vi "VILab.vi"() -> ()   [LabVIEW 2023, in "VILab.lvlib"]
uses:
  VILab.lvlib
  Support Files/VILab/VILab Data.ctl
  Support Files/VILab/Attribute.lvclass
  Resource Manipulation/Resource Array.ctl
  Resource Manipulation/Resource.ctl
  Support Files/VILab/Tree Manager.lvclass
  Support Files/VILab/State Enum.ctl
  Resource Manipulation/Decompose VI (Refnum).vi
  Support Files/VILab/Data Item.lvclass
  Resource Manipulation.lvlib
panel:
  in  "Dissect":bool
  in  "Rebuild":bool
  in  "Properties":bool
  in  "Clone":bool
  in  "Delete":bool
  in  "Add":bool
  in  "Tree":string(tree)
  # "WARNING:\nThis unofficial utility has NO WARRANTY and uses internal LabVIEW functionality that is NOT supported by National Instruments.\nYou will very likely crash LabVIEW and create insane/corrupted VI's, so use this at your own risk. But that's all part of the Fun™, right? ;)"
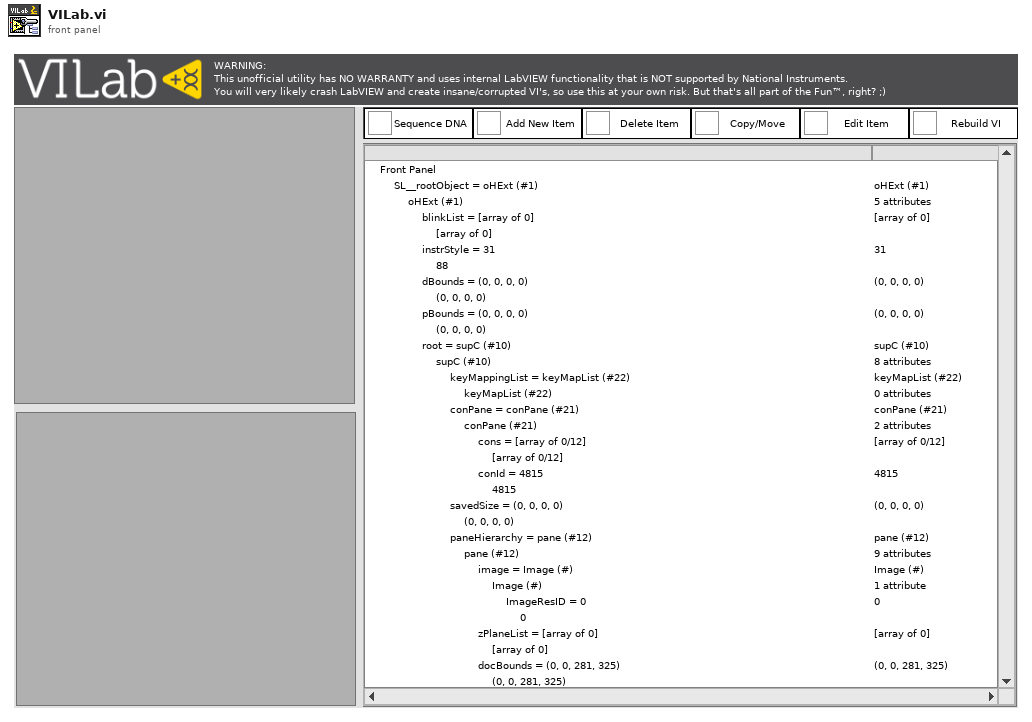
[diagram p1: front panel]
types:
  T1 = typedef "VILab.lvlib/State Enum.ctl" = enum16{"Initialize", "Event Handler", "Exit", "Edit Selected Item", "Dissect VI", "Rebuild VI"}
  T2 = typedef "VILab.lvlib/VILab Data.ctl" = cluster{"Embedded VI":refnum<vi>, "FP Root":refnum<class "Attribute.lvclass">, "BD Root":refnum<class "Attribute.lvclass">, "Def VI Res":T3, "Tree Mgr":refnum<class "Tree Manager.lvclass">}
  T3 = typedef "Resource Manipulation.lvlib/Resource Array.ctl" = T4[]
  T4 = typedef "Resource Manipulation.lvlib/Resource.ctl" = cluster{"type":u32, "id":i32, "name":string, "binary data":string}
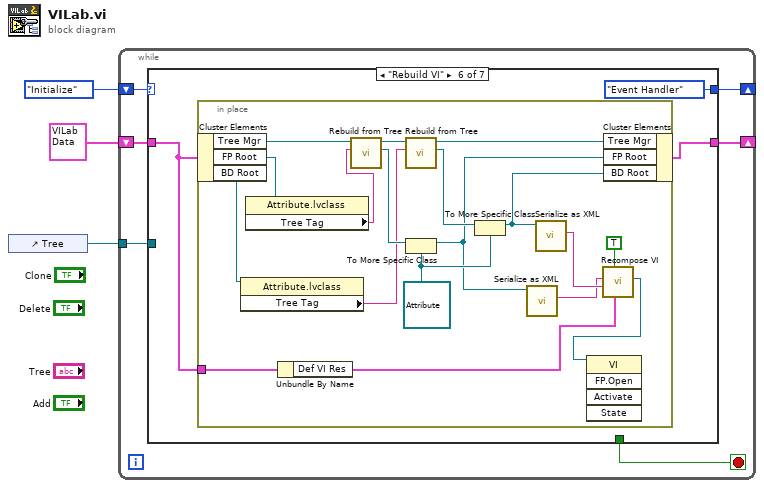
[diagram p0: block diagram]
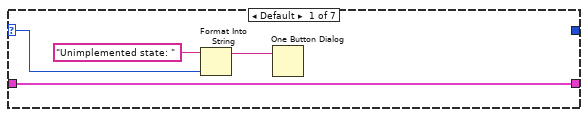
[diagram p2: hidden frame]
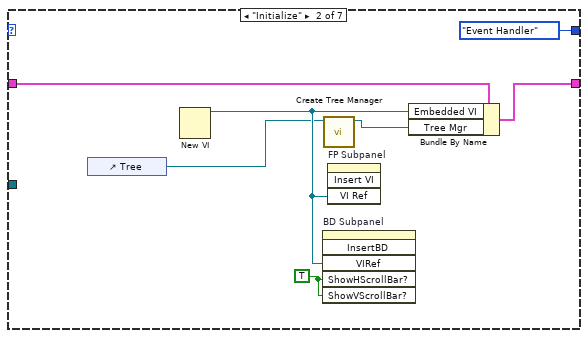
[diagram p3: hidden frame]
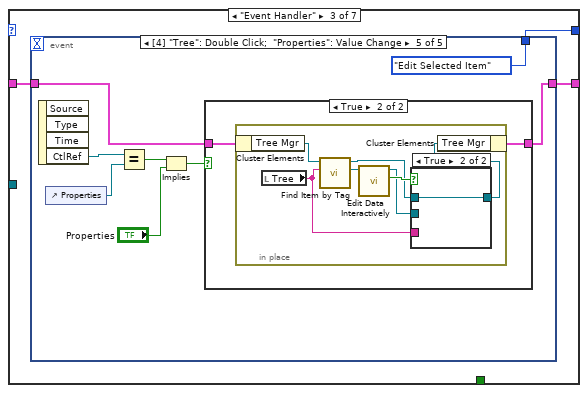
[diagram p4: hidden frame]
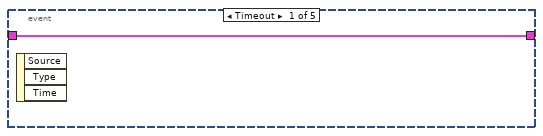
[diagram p5: hidden frame]
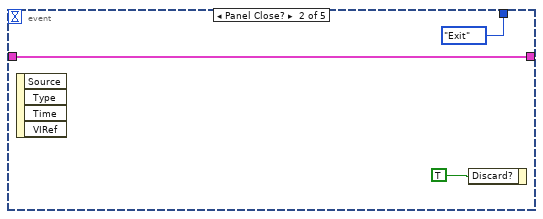
[diagram p6: hidden frame]
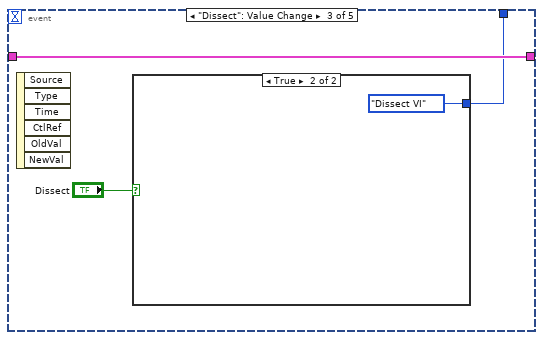
[diagram p7: hidden frame]
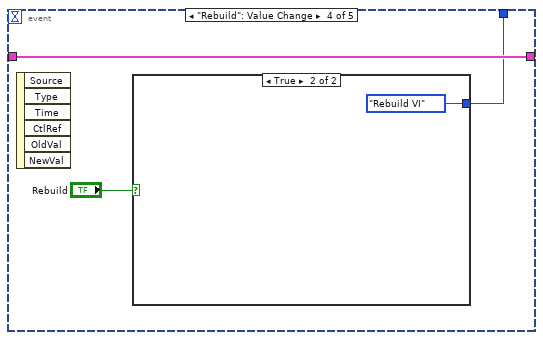
[diagram p9: hidden frame]
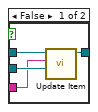
[diagram p12: hidden frame]
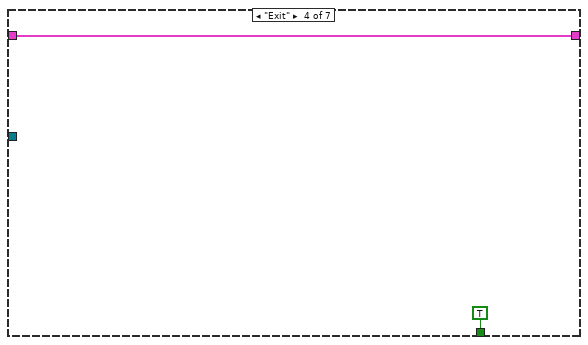
[diagram p13: hidden frame]
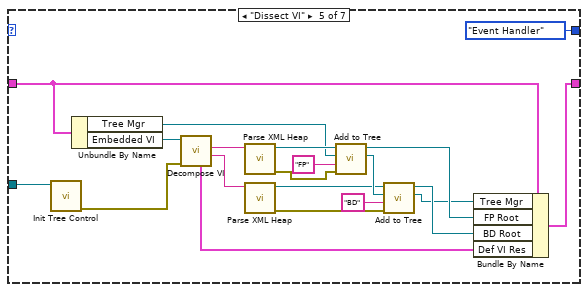
[diagram p14: hidden frame]
diagram:
  n1 = control-ref of="Tree"() -> (w1:refnum<vi>)
  n2 = while {
    shift-right: [w6] -> _
    shift-left: State_Enum."Initialize" ("State") -> [w9]
    shift-right: [w7] -> _
    shift-left: T2 {"Embedded VI"=refnum, "FP Root"=refnum, "BD Root"=refnum, "Def VI Res"=[], "Tree Mgr"=refnum} ("Data") -> [w8]
    tunnel: w1 -> [w4]
    stop <- w5 stop-if-true
    n3 = case shown="\"Rebuild VI\"" w9 {
      selector: w9 -> [w11 _ _ _ _ _ _]
      tunnel: w8 -> [w13 w20 w22 w60 w78 w81 w102]
      tunnel: [w13 w19 w23 w60 w76 w82 w102] -> w7
      tunnel: [_ State_Enum."Event Handler" ("State") w21 _ State_Enum."Event Handler" ("State") State_Enum."Event Handler" ("State") _] -> w6
      tunnel: [_ _ _ TRUE ("Discard?") _ _ _] -> w5
      tunnel: w4 -> [_ _ _ _ w65 _ _]
      frame Default {
        n4 = Format Into String(initial string="Unimplemented state: ", w11) -> (resulting string=w10:string)  [unwired: 2 in, 1 out]
        n5 = One Button Dialog(message=w10) -> ()  [unwired: 1 in, 1 out]
      }
      frame "Initialize" {
        w18 = TRUE ("ShowHScrollBar")
        n6 = control-ref of="Tree"() -> (w14:refnum<vi>)
        n7 = New VI() -> (3:w17:refnum<vi>)  [unwired: 7 in, 1 out]
        n8 = invoke on="BD Subpanel" class="SubPnl" method="InsertBD"("VIRef"=w17, "ShowHScrollBar?"=w18, "ShowVScrollBar?"=w18) -> ()  [unwired: 3 in, 6 out]
        n9 = call "Create Tree Manager.vi"("Tree Control"=w14) -> ("Tree Manager"=w15:refnum<class "Tree Manager.lvclass">)  [unwired: 9 in, 1 out]
        n10 = invoke on="FP Subpanel" class="SubPnl" method="Insert VI"("VI Ref"=w17) -> ()  [unwired: 3 in, 4 out]
        n11 = Bundle By Name(cluster=w20, "Embedded VI"=w17, "Tree Mgr"=w15) -> (w19:T2)
      }
      frame "Event Handler" {
        n12 = event shown="[4] \"Tree\": Double Click;  \"Properties\": Value Change" {
          selector: _ -> [_ _ _ _ _]
          dyn-events: _ -> [_ _ _ _ _]
          timeout: _ -> [_ _ _ _ _]
          tunnel: [w24 w27 w30 w34 w36] -> w23
          tunnel: w22 -> [w24 w27 w30 w34 w37]
          tunnel: [_ State_Enum."Exit" ("State") w28 w33 State_Enum."Edit Selected Item" ("State")] -> w21
          event Timeout {
            n13 = event-data() -> ()  [unwired: 1 in, 3 out]
          }
          event Panel Close? {
            n14 = event-data() -> ()  [unwired: 1 in, 4 out]
            n15 = event-data("Discard?"=TRUE) -> ()  [unwired: 1 in, 1 out]
          }
          event "Dissect": Value Change {
            n16 = event-data() -> ()  [unwired: 1 in, 6 out]
            n17 = case shown="True" "Dissect" {
              tunnel: [_ State_Enum."Dissect VI" ("State")] -> w28
              frame False {
              }
              frame True {
              }
            }
          }
          event "Rebuild": Value Change {
            n18 = event-data() -> ()  [unwired: 1 in, 6 out]
            n19 = case shown="True" "Rebuild" {
              tunnel: [_ State_Enum."Rebuild VI" ("State")] -> w33
              frame False {
              }
              frame True {
              }
            }
          }
          event "Tree": Double Click; "Properties": Value Change {
            n20 = event-data() -> ("CtlRef"=w42:refnum<vi>)  [unwired: 1 in, 3 out]
            n21 = control-ref of="Properties"() -> (w41:refnum<vi>)
            n22 = Equal?(x=w42, y=w41) -> (x = y?=w40:bool)
            n23 = Implies(1:"Properties", 2:w40) -> (0:w38:bool)
            n24 = case shown="True" w38 {
              tunnel: w37 -> [w44 w46]
              tunnel: [w44 w45] -> w36
              frame False {
              }
              frame True {
                n25 = in-place {
                  n26 = in-place-cluster #1(w46) -> ("Tree Mgr"=w52:refnum<class "Tree Manager.lvclass">)
                  n27 = local read "Tree"() -> (w47:string)
                  n28 = call "Find Item by Tag.vi"("Tag"=w47, "Tree Manager in"=w52) -> ("Data Item"=w53:refnum<class "Data Item.lvclass">, "Tree Manager out"=w49:refnum<class "Tree Manager.lvclass">)  [unwired: 6 in, 2 out]
                  n29 = call-dynamic "Edit Data Interactively.vi"("Data Item in"=w53) -> ("Cancel?"=w51:bool, "Data Item out"=w50:refnum<class "Data Item.lvclass">)  [unwired: 8 in, 1 out]
                  n30 = case shown="True" w51 {
                    tunnel: w50 -> [w57 _]
                    tunnel: w49 -> [w56 w58]
                    tunnel: [w55 w58] -> w48
                    tunnel: w47 -> [w54 _]
                    frame False {
                      n31 = call "Update Item.vi"("New Item"=w57, "Tag"=w54, "Tree Manager in"=w56) -> ("Tree Manager out"=w55:refnum<class "Tree Manager.lvclass">)  [unwired: 7 in, 1 out]
                    }
                    frame True {
                    }
                  }
                  n32 = in-place-cluster #1("Tree Mgr"=w48) -> (w45:T2)
                }
              }
            }
          }
        }
      }
      frame "Exit" {
      }
      frame "Dissect VI" {
        n33 = call "Init Tree Control.vi"("TreeControl in"=w65) -> ("Error out"=w64:errorcluster)  [unwired: 9 in, 1 out]
        n34 = Unbundle By Name(w78) -> ("Tree Mgr"=w73:refnum<class "Tree Manager.lvclass">, "Embedded VI"=w79:refnum<vi>)
        n35 = call-poly "Decompose VI.vi"("Error in"=w64, "VI Refnum"=w79) -> ("Block Diagram XML"=w63:string, "Front Panel XML"=w61:string, "Other resources"=w77:T3)  [unwired: 5 in, 2 out]
        n36 = call "Parse XML Heap.vi"("XML"=w61) -> ("Error out"=w72:errorcluster, "Root Element"=w75:refnum<class "Attribute.lvclass">)  [unwired: 9 in]
        n37 = call "Parse XML Heap.vi"("XML"=w63) -> ("Error out"=w71:errorcluster, "Root Element"=w62:refnum<class "Attribute.lvclass">)  [unwired: 9 in]
        n38 = call-dynamic "Add to Tree.vi"("error in (no error)"=w72, "Parent Tag"="FP", "Tree Manager in"=w73, "Attribute in"=w75) -> ("Tree Manager out"=w68:refnum<class "Tree Manager.lvclass">, "Attribute out"=w69:refnum<class "Attribute.lvclass">)  [unwired: 5 in, 1 out]
        n39 = call-dynamic "Add to Tree.vi"("error in (no error)"=w71, "Parent Tag"="BD", "Tree Manager in"=w68, "Attribute in"=w62) -> ("Tree Manager out"=w66:refnum<class "Tree Manager.lvclass">, "Attribute out"=w67:refnum<class "Attribute.lvclass">)  [unwired: 5 in, 1 out]
        n40 = Bundle By Name(cluster=w78, "Tree Mgr"=w66, "FP Root"=w69, "BD Root"=w67, "Def VI Res"=w77) -> (w76:T2)
      }
      frame "Rebuild VI" {
        n41 = in-place {
          in-place-border: w81 -> [w85]
          w97 = refnum<class "Attribute.lvclass"> refnum ("VILab.lvlib:Attribute.lvclass")
          n42 = in-place-cluster #2(w81) -> ("Tree Mgr"=w101:refnum<class "Tree Manager.lvclass">, "FP Root"=w91:refnum<class "Attribute.lvclass">, "BD Root"=w89:refnum<class "Attribute.lvclass">)
          n43 = property class="Attribute.lvclass"(reference=w89) -> ("Tree Tag"=w88:string)  [unwired: 1 in, 2 out]
          n44 = property class="Attribute.lvclass"(reference=w91) -> ("Tree Tag"=w90:string)  [unwired: 1 in, 2 out]
          n45 = Unbundle By Name(w85) -> ("Def VI Res"=w84:T3)
          n46 = call "Rebuild from Tree.vi"("Tag"=w90, "Tree Manager in"=w101) -> ("Rebuilt Item"=w99:refnum<class "Data Item.lvclass">, "Tree Manager out"=w100:refnum<class "Tree Manager.lvclass">)  [unwired: 7 in, 1 out]
          n47 = call "Rebuild from Tree.vi"("Tag"=w88, "Tree Manager in"=w100) -> ("Rebuilt Item"=w98:refnum<class "Data Item.lvclass">, "Tree Manager out"=w96:refnum<class "Tree Manager.lvclass">)  [unwired: 7 in, 1 out]
          n48 = To More Specific Class(target class=w97, reference=w99) -> (specific class reference=w94:refnum<class "Attribute.lvclass">)  [unwired: 1 in, 1 out]
          n49 = To More Specific Class(target class=w97, reference=w98) -> (specific class reference=w95:refnum<class "Attribute.lvclass">)  [unwired: 1 in, 1 out]
          n50 = call-dynamic "Serialize as XML.vi"("Attribute in"=w94) -> ("XML Fragment"=w86:string)  [unwired: 8 in, 2 out]
          n51 = call-dynamic "Serialize as XML.vi"("Attribute in"=w95) -> ("XML Fragment"=w87:string)  [unwired: 8 in, 2 out]
          n52 = call "Recompose VI.vi"("Other resources (default)"=w84, "Open VI? (F)"=TRUE, "Block Diagram XML"=w87, "Front Panel XML"=w86) -> ("VI Refnum (if opened)"=w93:refnum<vi>)  [unwired: 5 in, 2 out]
          n53 = invoke class="VI" method="FP.Open"(reference=w93) -> ()  [unwired: 4 in, 5 out]
          n54 = in-place-cluster #2("Tree Mgr"=w96, "FP Root"=w94, "BD Root"=w95) -> (w82:T2)
        }
      }
      frame "Edit Selected Item" {
      }
    }
  }
